vi "Read Attributes.vi"(11 "RTM Activated Msg":refnum<class "RTM Activated Msg.lvclass">) -> (2 "Payload":cluster{"Tag":string, "VI Name":string})   [LabVIEW 2015, in "Interface.lvlib" / "RTM Activated Msg.lvclass"]
uses:
  RTM Activated Msg.lvclass
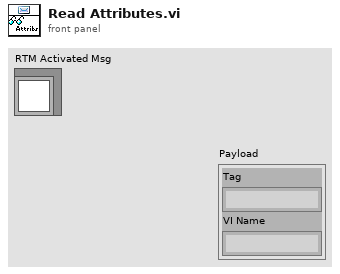
[diagram p1: front panel]
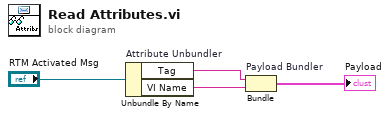
[diagram p0: block diagram]
diagram:
  n1 = Unbundle By Name "Attribute Unbundler"("RTM Activated Msg") -> ("Tag"=w2:string, "VI Name"=w1:string)
  n2 = Bundle "Payload Bundler"("Tag"=w2, "VI Name"=w1) -> (→"Payload":cluster{"Tag":string, "VI Name":string})  [unwired: 1 in]
